vi "getResponse.vi"(8 "error in (no error)":errorcluster, 9 "Function":u8, 10 "Address":u8, 11 "Mockbus in":refnum<class "Mockbus.lvclass">) -> (0 "error out":errorcluster, 2 "Frame":T1 {"Data" format="%02x"}, 3 "Mockbus out":refnum<class "Mockbus.lvclass">)   [LabVIEW 2016, in "RTMockbus.lvlib" / "Mockbus.lvclass"]
uses:
  Mockbus.lvclass
  Common_RT_Modbus/DataTypes/TxFrame.ctl
  Mockbus.lvclass/Mockbus.ctl
  Common_RT_Modbus/DynamicFrameBuilder/DynamicFrameBuilder.lvclass
  Common_RT_Modbus/RTModbus.lvlib
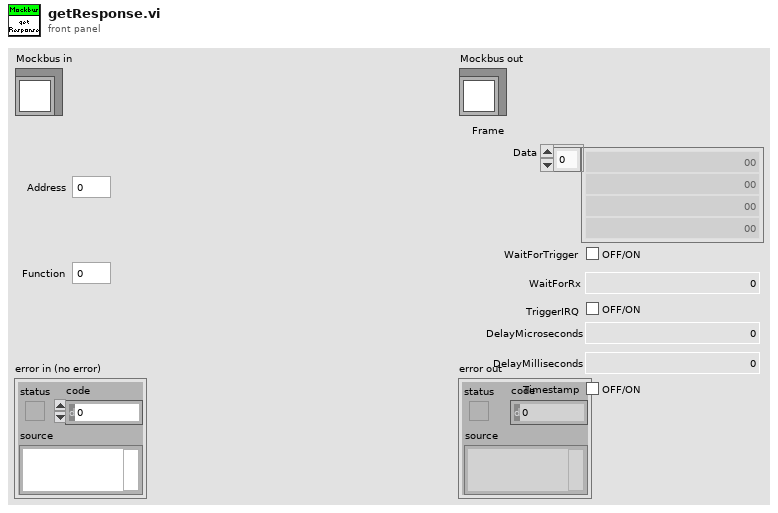
[diagram p1: front panel]
types:
  T1 = typedef "RTModbus.lvlib/TxFrame.ctl" = cluster{"Data":u8[], "WaitForTrigger":bool, "WaitForRx":u16, "TriggerIRQ":bool, "DelayMicroseconds":u16, "DelayMilliseconds":u16, "Timestamp":bool}
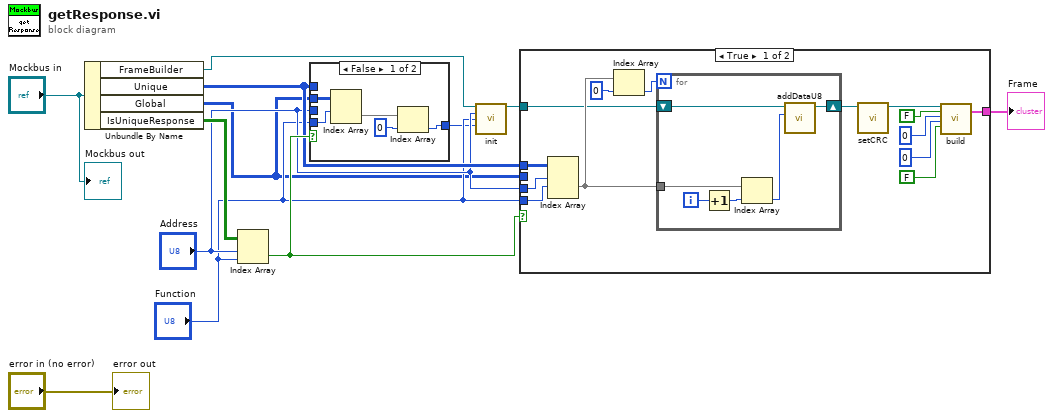
[diagram p0: block diagram]
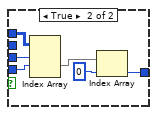
[diagram p2: hidden frame]
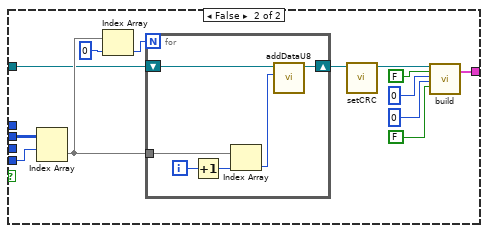
[diagram p3: hidden frame]
diagram:
  n1 = Unbundle By Name("Mockbus in") -> ("FrameBuilder"=w8:refnum<class "DynamicFrameBuilder.lvclass">, "Unique"=w5:u8[][][], "Global"=w2:u8[][], "IsUniqueResponse"=w10:bool[][])
  n2 = Index Array(array=w10, index (row)="Address", index (col)="Function") -> (element=w6:bool)
  n3 = case shown="False" w6 {
    tunnel: w5 -> [_ w23]
    tunnel: "Address" -> [_ w22]
    tunnel: "Function" -> [w14 w21]
    tunnel: [w13 w18] -> w1
    tunnel: w2 -> [w15 _]
    frame False {
      n4 = Index Array(array=w15, index (row)=w14) -> (element=w16:u8[])  [unwired: 1 in]
      n5 = Index Array(array=w16, index=0) -> (element=w13:u8)
    }
    frame True {
      n6 = Index Array(array=w23, index (dim 0)=w22, index (dim 1)=w21) -> (element=w19:u8[])  [unwired: 1 in]
      n7 = Index Array(array=w19, index=0) -> (element=w18:u8)
    }
  }
  n8 = call "init.vi"("DynamicFrameBuilder in"=w8, "Address"="Address", "Function"="Function", "DataSize"=w1) -> ("DynamicFrameBuilder out"=w7:refnum<class "DynamicFrameBuilder.lvclass">)  [unwired: 10 in, 1 out]
  n9 = case shown="True" w6 {
    tunnel: w2 -> [_ w56]
    tunnel: "Function" -> [w36 w52]
    tunnel: w5 -> [w37 _]
    tunnel: "Address" -> [w32 _]
    tunnel: w7 -> [w31 w51]
    tunnel: [w28 w48] -> w9
    frame True {
      n10 = Index Array(array=w37, index (dim 0)=w32, index (dim 1)=w36) -> (element=w33:u8[])  [unwired: 1 in]
      n11 = Index Array(array=w33, index=0) -> (element=w34:u8)
      n12 = for {
        N: w34 -> [_]
        tunnel: w33 -> [w43]
        shift-right: [w38] -> w30
        shift-left: w31 -> [w39]
        i -> [w42]
        n13 = Increment(x=w42) -> (x+1=w41:i32)
        n14 = Index Array(array=w43, index=w41) -> (element=w40:u8)
        n15 = call "addDataU8.vi"("Data"=w40, "DynamicFrameBuilder in"=w39) -> ("DynamicFrameBuilder out"=w38:refnum<class "DynamicFrameBuilder.lvclass">)  [unwired: 8 in, 1 out]
      }
      n16 = call "setCRC.vi"("DynamicFrameBuilder in"=w30) -> ("DynamicFrameBuilder out"=w29:refnum<class "DynamicFrameBuilder.lvclass">)  [unwired: 9 in, 1 out]
      n17 = call "build.vi"("DynamicFrameBuilder in"=w29, "WaitForTrigger"=FALSE ("WaitForTrigger?"), "Latency"=u32 0, "WaitForRxTimeout"=u16 0, "TriggerIRQ"=FALSE ("TriggerIRQ?")) -> ("TxFrame"=w28:T1)  [unwired: 12 in, 2 out]
    }
    frame False {
      n18 = Index Array(array=w56, index (row)=w52) -> (element=w53:u8[])  [unwired: 1 in]
      n19 = Index Array(array=w53, index=0) -> (element=w54:u8)
      n20 = for {
        N: w54 -> [_]
        tunnel: w53 -> [w60]
        shift-right: [w57] -> w50
        shift-left: w51 -> [w58]
        i -> [w62]
        n21 = Increment(x=w62) -> (x+1=w61:i32)
        n22 = Index Array(array=w60, index=w61) -> (element=w59:u8)
        n23 = call "addDataU8.vi"("Data"=w59, "DynamicFrameBuilder in"=w58) -> ("DynamicFrameBuilder out"=w57:refnum<class "DynamicFrameBuilder.lvclass">)  [unwired: 8 in, 1 out]
      }
      n24 = call "setCRC.vi"("DynamicFrameBuilder in"=w50) -> ("DynamicFrameBuilder out"=w49:refnum<class "DynamicFrameBuilder.lvclass">)  [unwired: 9 in, 1 out]
      n25 = call "build.vi"("DynamicFrameBuilder in"=w49, "WaitForTrigger"=FALSE ("WaitForTrigger?"), "Latency"=u32 0, "WaitForRxTimeout"=u16 0, "TriggerIRQ"=FALSE ("TriggerIRQ?")) -> ("TxFrame"=w48:T1)  [unwired: 12 in, 2 out]
    }
  }
  "Frame" <- w9
  "error out" <- "error in (no error)"
  "Mockbus out" <- "Mockbus in"
